vi "OnActivate.vi"(8 "Error In":errorcluster, 11 "reference in":refnum<class "FlyingEnchantment.lvclass">) -> (0 "Error Out":errorcluster, 3 "reference out":refnum<class "FlyingEnchantment.lvclass">)   [LabVIEW 2020, in "FlyingEnchantment.lvclass"]
uses:
  FlyingEnchantment.lvclass
  Console_class/Console.lvclass
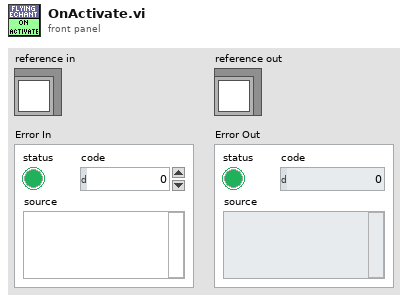
[diagram p1: front panel]
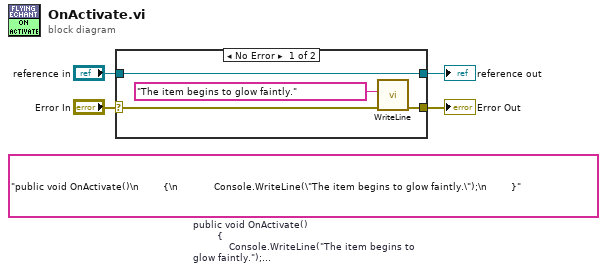
[diagram p0: block diagram]
diagram:
  (unwired) "public void OnActivate()\n        {\n            Console.WriteLine(\"The item begins to glow faintly.\");\n        }"  # public void OnActivate()         {             Console.WriteLine("The item begins to glow faintly.");         }
  n1 = case shown="No Error" "Error In" {
    selector: "Error In" -> [w7 w10]
    tunnel: [w6 w10] -> w3
    tunnel: [w8 w9] -> w1
    tunnel: "reference in" -> [w8 w9]
    frame No Error {
      n2 = call "WriteLine.vi"("Error In"=w7, "ConsoleText"="The item begins to glow faintly.") -> ("Error Out"=w6:errorcluster)  [unwired: 9 in]
    }
    frame Error {
    }
  }
  "Error Out" <- w3
  "reference out" <- w1
